vi "NI 9208 Getting Started (FPGA).vi"() -> ()   [LabVIEW 2015]
doc: "This VI continually reads single point values from all 16 channels of the NI 9208."
uses:
  <vilib>/LabVIEW Targets/FPGA/cRIO/shared/nicrio_ModuleControls/nicrio_BasicConversionTime.ctl
  <vilib>/rvi/Emulation/niFpgaGetClockAttributes.vi
  <vilib>/rvi/Emulation/niFpgaSctlEmulationGetInTimedLoop.vi
  <vilib>/rvi/Emulation/niFpgaEmulationReportErrorSimple.vi
  <vilib>/rvi/eio/common/nirviEmuTemplatePropertySet_errors.vi
  <vilib>/rvi/eio/common/nirviEmuTemplateMethod_errors.vi
  <vilib>/rvi/Emulation/niFpgaCriticalErrorInLSC.vi
  <vilib>/eio/EIOPropertyNode/EIOPropertyNode.xnode
  <vilib>/eio/EIONode/EIONode.xnode
  <vilib>/rvi/eio/common/nirviEmuTemplatePropertyGet_errors.vi
  <vilib>/rvi/eio/common/nirviEmuTemplatePropertyGet_noerrors.vi
  <vilib>/rvi/eio/common/nirviEmuTemplatePropertySet_noerrors.vi
panel:
  out "Current Data":fxp<+/-,24,-4>[](array[numeric]) format="%.27g"
  out "FPGA Error Out":errorcluster
  in  "Conversion Time":T1=enum."High Resolution"
  in  "Update Conversion Time":bool
  in  "Stop":bool
  # "Overview: Demonstrates how to acquire data from the NI 9208\nRequirements: LabVIEW Full Development System, LV FPGA, and NI RIO\nInstructions: \n1. Run NI 9208 Getting Started (Host).vi"
  # "Current Data"
  # "Error Cluster"
  # "Input Parameters"
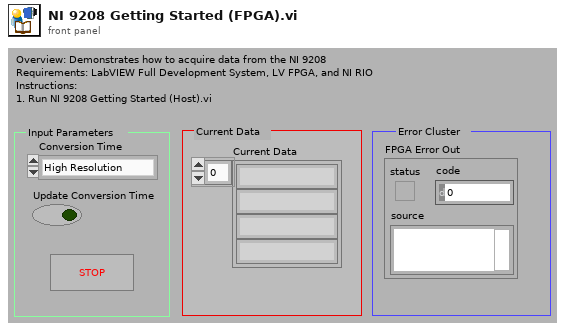
[diagram p1: front panel]
types:
  T1 = typedef "nicrio_BasicConversionTime.ctl" = enum8{"High Speed", "High Resolution"}
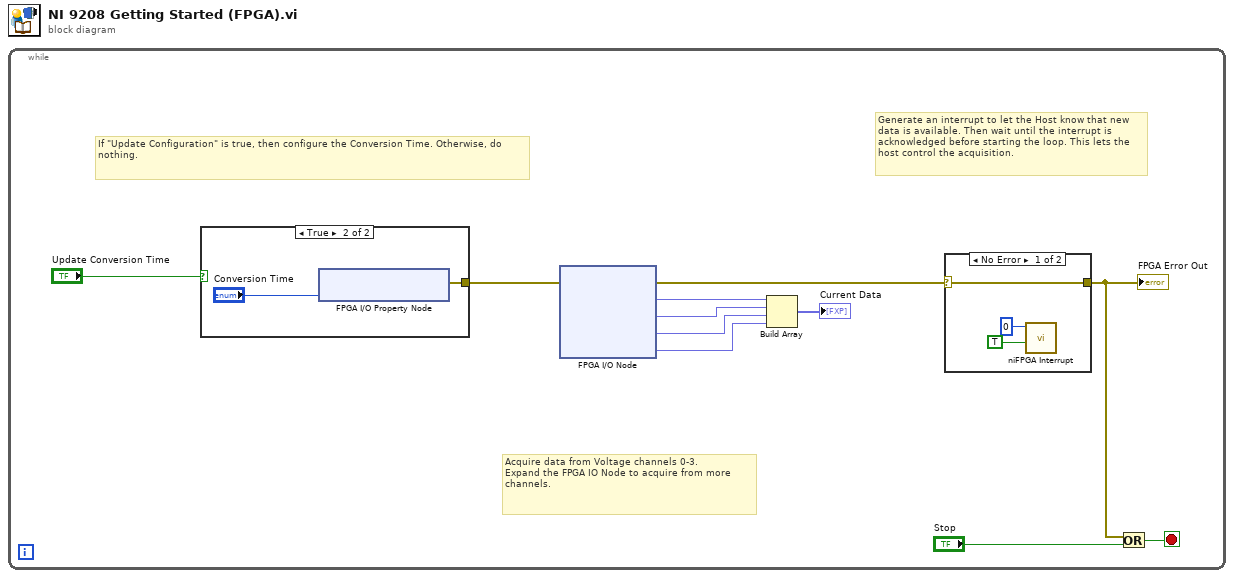
[diagram p0: block diagram]
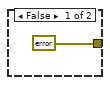
[diagram p3: hidden frame]
diagram:
  n1 = while {
    stop <- w6 stop-if-true
    # "If \"Update Configuration\" is true, then configure the Conversion Time. Otherwise, do nothing."
    # "Acquire data from Voltage channels 0-3. \nExpand the FPGA IO Node to acquire from more channels."
    # "Generate an interrupt to let the Host know that new data is available. Then wait until the interrupt is acknowledged before starting the loop. This lets the host control the acquisition."
    n2 = case shown="True" "Update Conversion Time" {
      tunnel: [errorcluster {"status"=FALSE, "code"=0, "source"=""} ("error out") w18] -> w11
      frame False {
      }
      frame True {
        n3 = xnode "FPGA I/O Property Node"("Conversion Time"="Conversion Time") -> ("error out"=w18:errorcluster)  [unwired: 2 in, 1 out]
      }
    }
    n4 = xnode "FPGA I/O Node"("error in"=w11) -> ("error out"=w5:errorcluster, "Mod1/AI0"=w10:fxp<+/-,24,4>, "Mod1/AI1"=w9:fxp<+/-,24,4>, "Mod1/AI2"=w8:fxp<+/-,24,4>, "Mod1/AI3"=w7:fxp<+/-,24,4>)  [unwired: 4 in, 4 out]
    n5 = Build Array(w10, w9, w8, w7) -> (→"Current Data":fxp<+/-,24,4>[])
    n6 = case shown="No Error" w5 {
      selector: w5 -> [w12 w15]
      tunnel: [w12 w15] -> w1
      frame No Error {
        n7 = call <vilib>:"niFPGA Interrupt.vi"("Wait Until Cleared (F)"=TRUE ("Wait Until Cleared"), "IRQ Number (0)"=u8 0 ("IRQ Bit (0-31)")) -> ()  [unwired: 1 in]
      }
      frame Error {
      }
    }
    "FPGA Error Out" <- w1
    n8 = Or(x=w1, y="Stop") -> (x .or. y?=w6:bool)
  }
